vi "Recursive Search Owned Items for XML files.vi"(8 "error in (no error)":errorcluster, 11 "Owned Items[]":refnum<vi>[](array[refnum])) -> (0 "error out":errorcluster, 2 "xml files found":path[](array[path]))   [LabVIEW 2019, in "Configuration Tool.lvlib"]
uses:
  Configuration Tool.lvlib
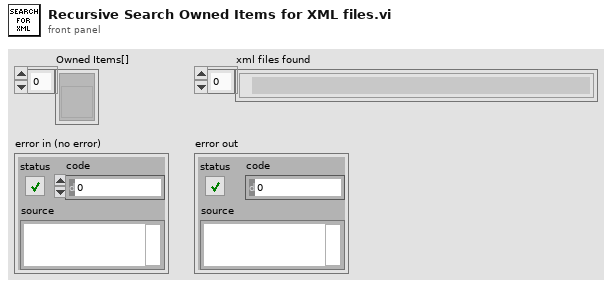
[diagram p1: front panel]
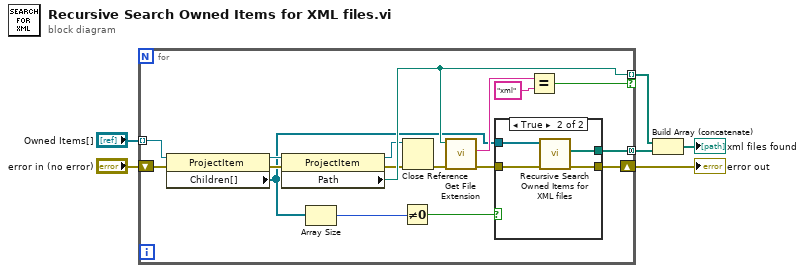
[diagram p0: block diagram]
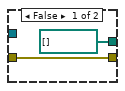
[diagram p2: hidden frame]
diagram:
  n1 = for {
    tunnel: "Owned Items[]" -> [w23] mode=indexing
    tunnel: [w20] -> w6 mode=indexing if=w17
    tunnel: [w14] -> w5 mode=concatenating
    shift-right: [w10] -> w1
    shift-left: "error in (no error)" -> [w12]
    n2 = property class="ProjectItem"(reference=w23, error in=w12) -> (reference out=w22:refnum<vi>, error out=w21:errorcluster, "Children[]"=w13:refnum<vi>[])
    n3 = property class="ProjectItem"(reference=w22, error in=w21) -> (reference out=w9:refnum<vi>, error out=w8:errorcluster, "Path"=w20:path)
    n4 = Array Size(array=w13) -> (size(s)=w16:i32)
    n5 = Not Equal To 0?(x=w16) -> (x != 0?=w15:bool)
    n6 = Close Reference(reference=w9, error in (no error)=w8) -> (error out=w7:errorcluster)
    n7 = call <vilib>:"Get File Extension.vi"("error in (no error)"=w7, "file"=w20) -> ("error out"=w11:errorcluster, "lowercase file extension"=w19:string)  [unwired: 5 in, 3 out]
    n8 = case shown="True" w15 {
      tunnel: w13 -> [_ w29]
      tunnel: [path[] [] ("xml files found") w28] -> w14
      tunnel: w11 -> [w24 w27]
      tunnel: [w24 w26] -> w10
      frame False {
      }
      frame True {
        n9 = call "Recursive Search Owned Items for XML files.vi"("error in (no error)"=w27, "Owned Items[]"=w29) -> ("error out"=w26:errorcluster, "xml files found"=w28:path[])  [unwired: 8 in]
      }
    }
    n10 = Equal?(x=w19, y="xml") -> (x = y?=w17:bool)
  }
  "error out" <- w1
  n11 = Build Array (concatenate)(w6, w5) -> (→"xml files found":path[])
